vi "Create.vi"(8 "error in (no error)":errorcluster) -> (0 "error out":errorcluster, 3 "Event Registration Refnum":refnum<event-registration>)   [LabVIEW 2017, in "WebServiceImporter.lvlib" / "Main Panel.lvlib" / "Input Info.lvlib" / "Events.lvlib"]
uses:
  <vilib>/Platform/WebService/Main Panel/Pages/Input Info/Events/Events.lvlib
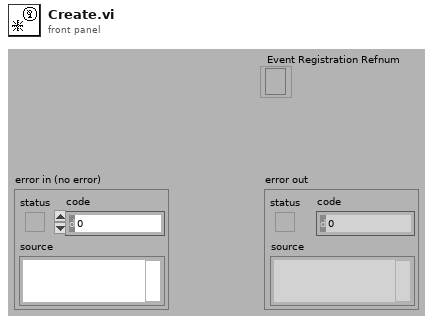
[diagram p1: front panel]
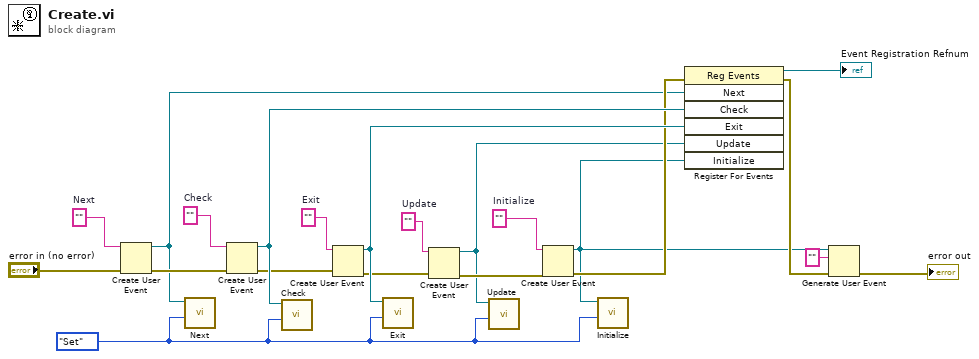
[diagram p0: block diagram]
diagram:
  w5 = ""  # Next
  w7 = ""  # Update
  w17 = ""  # Initialize
  w19 = ""  # Exit
  w1 = enum16{"Get", "Set"}."Set" ("Operation")
  w21 = ""  # Check
  n1 = Create User Event(user event datatype=w5, error in="error in (no error)") -> (user event=w2:refnum<user-event>, error out=w3:errorcluster)
  n2 = call <vilib>:"Next.vi"("Operation"=w1, "user event"=w2) -> ()  [unwired: 9 in, 1 out]
  n3 = Create User Event(user event datatype=w21, error in=w3) -> (user event=w20:refnum<user-event>, error out=w18:errorcluster)
  n4 = call <vilib>:"Check.vi"("Operation"=w1, "user event"=w20) -> ()  [unwired: 8 in, 2 out]
  n5 = Create User Event(user event datatype=w19, error in=w18) -> (user event=w16:refnum<user-event>, error out=w11:errorcluster)
  n6 = call <vilib>:"Exit.vi"("Operation"=w1, "user event"=w16) -> ()  [unwired: 8 in, 2 out]
  n7 = Create User Event(user event datatype=w7, error in=w11) -> (user event=w8:refnum<user-event>, error out=w10:errorcluster)
  n8 = call <vilib>:"Update.vi"("Operation"=w1, "user event"=w8) -> ()  [unwired: 8 in, 2 out]
  n9 = Create User Event(user event datatype=w17, error in=w10) -> (user event=w9:refnum<user-event>, error out=w15:errorcluster)
  n10 = call <vilib>:"Initialize.vi"("Operation"=w1, "user event"=w9) -> ()  [unwired: 9 in, 1 out]
  n11 = register-events(error in=w15, w2, w20, w16, w8, w9) -> (reference out=→"Event Registration Refnum":refnum<event-registration>, error out=w13:errorcluster)  [unwired: 1 in]
  n12 = Generate User Event(user event=w9, event data cluster="" ("event data"), error in=w13) -> (error out=→"error out":errorcluster)  [unwired: 1 in, 1 out]
